vi "Camera_Feed.vi"(8 "error in":errorcluster, 11 "DataCluster":T1={"Core"={"Current VI Reference"=refnum, "Close Panel on Exit?"=FALSE, "Exit"=FALSE, "Initialized?"=FALSE}, "Connections"={"cDAQ Therm"={"Task"="", "Connected"=FALSE, "Active"=FALSE}, "cDAQ Voltage"={"Task"="", "Connected"=FALSE, "Active"=FALSE}, "cDAQ ID"="", "Camera"={"Session"="", "Connected"=FALSE, "Active"=FALSE, "Placeholder"=refnum}, "PSU"={"Port"="", "Connected"=FALSE, "Active"=FALSE}}, "Data Acquisition"={"Setup"={"Label"="", "Operator"="", "Notes"="", "TempGrad"=0.0, "TargetTemp"=0.0, "Sample Volume"=1.0}, "Camera"={"Image"=refnum, "Save Image"=refnum, "Image Frequency"=20, "Rectangle"={"Left"=0, "Top"=0, "Right"=0, "Bottom"=0, "Rotation"=0.0}, "Calibration"={"Top Left"={"X"=0.0, "Y"=0.0}, "Top Right"={"X"=0.0, "Y"=0.0}, "Bottom Left"={"X"=0.0, "Y"=0.0}, "Bottom Right"={"X"=0.0, "Y"=0.0}, "Fixpoint"={"X"=0.0, "Y"=0.0}, "Scan Area"=0.0, "Fixpoint Area"=0.0, "Well Pixels"=[], "Valid"=FALSE}, "FocusPos"=0, "Display Mapping"=10}, "Thermistor"={"Sample Size"=0, "Calibration"={"B0.100"=[], "R25"=[], "c"=[], "State"=[], "V_S"=0.0, "R_S"=0.0}, "Timing Mode"=14713}, "Partition"={"Data"=[], "Cell Label"="", "Cell Color"=0, "Height"=10, "Width"=16, "Grid"=[]}, "Queue"={"Size"=0, "Queue"=refnum}, "Sample Rate"=0, "Active"=FALSE, "Ready"=FALSE, "Graph Mode"=0}, "Control"={"Sample Rate"=0, "PID gains"={"proportional gain (Kc)"=0.0, "integral time (Ti, min)"=0.0, "derivative time (Td, min)"=0.0}}} {"Control"."PID gains"."derivative time (Td, min)" format="%.3f"; "Control"."PID gains"."integral time (Ti, min)" format="%.3f"; "Control"."PID gains"."proportional gain (Kc)" format="%.3f"; "Control"."Sample Rate" min=1 max=20 step=1 format="%.0f Samples/sec"; "Data Acquisition"."Graph Mode" items=["Thermistor Temperature", "Camera Temperature"]; "Data Acquisition"."Thermistor"."Timing Mode" items=["Automatic"=16097, "High Resolution"=10195, "High Speed"=14712, "Best 50 Hz Rejection"=14713, "Best 60 Hz Rejection"=14714, "Custom"=10137]; "Data Acquisition"."Thermistor"."Calibration"."R_S" min=0.1 max=1000.0 format="%#_g kOhm"; "Data Acquisition"."Thermistor"."Calibration"."V_S" min=5.0 max=48.0 format="%#_g V"; "Data Acquisition"."Thermistor"."Calibration"."R25" min=0.1 max=1000.0 format="%#_g kOhm"; "Data Acquisition"."Thermistor"."Calibration"."B0.100" min=100.0 max=10000.0 format="%#_g K"; "Data Acquisition"."Thermistor"."Sample Size" min=1 max=200; "Data Acquisition"."Sample Rate" min=20 max=240 format="%.0f samples/min"; "Data Acquisition"."Queue"."Size" min=1 max=200; "Data Acquisition"."Camera"."Display Mapping" items=["Default"=10, "Most Significant Bits"=11, "Full Dynamic"=12, "Downshift"=13, "Given Range"=14, "90% Dynamic"=15, "Given Percent Range"=16]; "Data Acquisition"."Camera"."Calibration"."Fixpoint"."Y" format="%.2f"; "Data Acquisition"."Camera"."Calibration"."Fixpoint"."X" format="%.2f"; "Data Acquisition"."Camera"."Calibration"."Top Left"."Y" format="%.2f"; "Data Acquisition"."Camera"."Calibration"."Top Left"."X" format="%.2f"; "Data Acquisition"."Camera"."Calibration"."Top Right"."Y" format="%.2f"; "Data Acquisition"."Camera"."Calibration"."Top Right"."X" format="%.2f"; "Data Acquisition"."Camera"."Calibration"."Bottom Left"."Y" format="%.2f"; "Data Acquisition"."Camera"."Calibration"."Bottom Left"."X" format="%.2f"; "Data Acquisition"."Camera"."Calibration"."Bottom Right"."Y" format="%.2f"; "Data Acquisition"."Camera"."Calibration"."Bottom Right"."X" format="%.2f"; "Data Acquisition"."Camera"."Rectangle"."Rotation" min=-90.0 max=90.0 step=1.0 format="%.2f"; "Data Acquisition"."Camera"."Rectangle"."Left" scale=0.0..1024.0; "Data Acquisition"."Camera"."Rectangle"."Right" scale=0.0..1024.0; "Data Acquisition"."Camera"."Image Frequency" min=1 max=60 step=1; "Data Acquisition"."Setup"."Sample Volume" min=0.0 max=500.0 format="%#_g µL"; "Data Acquisition"."Setup"."TargetTemp" min=-40.0 max=40.0 step=0.5 format="%#_g °C"; "Data Acquisition"."Setup"."TempGrad" min=-100.0 max=100.0 step=0.1 format="%#_g °C/min"}) -> (0 "error out":errorcluster, 3 "DataCluster out":T1={"Core"={"Current VI Reference"=refnum, "Close Panel on Exit?"=FALSE, "Exit"=FALSE, "Initialized?"=FALSE}, "Connections"={"cDAQ Therm"={"Task"="", "Connected"=FALSE, "Active"=FALSE}, "cDAQ Voltage"={"Task"="", "Connected"=FALSE, "Active"=FALSE}, "cDAQ ID"="", "Camera"={"Session"="", "Connected"=FALSE, "Active"=FALSE, "Placeholder"=refnum}, "PSU"={"Port"="", "Connected"=FALSE, "Active"=FALSE}}, "Data Acquisition"={"Setup"={"Label"="", "Operator"="", "Notes"="", "TempGrad"=1.0, "TargetTemp"=1.0, "Sample Volume"=1.0}, "Camera"={"Image"=refnum, "Save Image"=refnum, "Image Frequency"=20, "Rectangle"={"Left"=0, "Top"=0, "Right"=0, "Bottom"=0, "Rotation"=0.0}, "Calibration"={"Top Left"={"X"=0.0, "Y"=0.0}, "Top Right"={"X"=0.0, "Y"=0.0}, "Bottom Left"={"X"=0.0, "Y"=0.0}, "Bottom Right"={"X"=0.0, "Y"=0.0}, "Fixpoint"={"X"=0.0, "Y"=0.0}, "Scan Area"=0.0, "Fixpoint Area"=0.0, "Well Pixels"=[], "Valid"=FALSE}, "FocusPos"=0, "Display Mapping"=10}, "Thermistor"={"Sample Size"=1, "Calibration"={"B0.100"=[], "R25"=[], "c"=[], "State"=[], "V_S"=5.0, "R_S"=100.0}, "Timing Mode"=14713}, "Partition"={"Data"=[], "Cell Label"="", "Cell Color"=0, "Height"=10, "Width"=16, "Grid"=[]}, "Queue"={"Size"=1, "Queue"=refnum}, "Sample Rate"=20, "Active"=FALSE, "Ready"=FALSE, "Graph Mode"=0}, "Control"={"Sample Rate"=1, "PID gains"={"proportional gain (Kc)"=1.0, "integral time (Ti, min)"=0.01, "derivative time (Td, min)"=0.0}}} {"Control"."PID gains"."derivative time (Td, min)" format="%.3f"; "Control"."PID gains"."integral time (Ti, min)" format="%.3f"; "Control"."PID gains"."proportional gain (Kc)" format="%.3f"; "Control"."Sample Rate" min=1 max=20 step=1 format="%.0f Samples/sec"; "Data Acquisition"."Graph Mode" items=["Thermistor Temperature", "Camera Temperature"]; "Data Acquisition"."Thermistor"."Timing Mode" items=["Automatic"=16097, "High Resolution"=10195, "High Speed"=14712, "Best 50 Hz Rejection"=14713, "Best 60 Hz Rejection"=14714, "Custom"=10137]; "Data Acquisition"."Thermistor"."Calibration"."R_S" min=0.1 max=1000.0 format="%#_g kOhm"; "Data Acquisition"."Thermistor"."Calibration"."V_S" min=5.0 max=48.0 format="%#_g V"; "Data Acquisition"."Thermistor"."Calibration"."R25" min=0.1 max=1000.0 format="%#_g kOhm"; "Data Acquisition"."Thermistor"."Calibration"."B0.100" min=100.0 max=10000.0 format="%#_g K"; "Data Acquisition"."Thermistor"."Sample Size" min=1 max=200; "Data Acquisition"."Sample Rate" min=20 max=240 format="%.0f samples/min"; "Data Acquisition"."Queue"."Size" min=1 max=200; "Data Acquisition"."Camera"."Display Mapping" items=["Default"=10, "Most Significant Bits"=11, "Full Dynamic"=12, "Downshift"=13, "Given Range"=14, "90% Dynamic"=15, "Given Percent Range"=16]; "Data Acquisition"."Camera"."Calibration"."Fixpoint"."Y" format="%.2f"; "Data Acquisition"."Camera"."Calibration"."Fixpoint"."X" format="%.2f"; "Data Acquisition"."Camera"."Calibration"."Top Left"."Y" format="%.2f"; "Data Acquisition"."Camera"."Calibration"."Top Left"."X" format="%.2f"; "Data Acquisition"."Camera"."Calibration"."Top Right"."Y" format="%.2f"; "Data Acquisition"."Camera"."Calibration"."Top Right"."X" format="%.2f"; "Data Acquisition"."Camera"."Calibration"."Bottom Left"."Y" format="%.2f"; "Data Acquisition"."Camera"."Calibration"."Bottom Left"."X" format="%.2f"; "Data Acquisition"."Camera"."Calibration"."Bottom Right"."Y" format="%.2f"; "Data Acquisition"."Camera"."Calibration"."Bottom Right"."X" format="%.2f"; "Data Acquisition"."Camera"."Rectangle"."Rotation" min=-90.0 max=90.0 step=1.0 format="%.2f"; "Data Acquisition"."Camera"."Rectangle"."Left" scale=0.0..1024.0; "Data Acquisition"."Camera"."Rectangle"."Right" scale=0.0..1024.0; "Data Acquisition"."Camera"."Image Frequency" min=1 max=60 step=1; "Data Acquisition"."Setup"."Sample Volume" min=0.0 max=500.0 format="%#_g µL"; "Data Acquisition"."Setup"."TargetTemp" min=-40.0 max=40.0 step=0.5 format="%#_g °C"; "Data Acquisition"."Setup"."TempGrad" min=-100.0 max=100.0 step=0.1 format="%#_g °C/min"})   [LabVIEW 2020]
uses:
  DataCluster.ctl
  <vilib>/userDefined/High Color/IMAQdx.ctl
  <vilib>/vision/Image Controls.llb/IMAQ Image.ctl
  <resource>/objmgr/imaqdx.rc
panel:
  out "Feed":T3(plugin-control) caption="Camera Feed"
  out "FocusPos":u32 caption="Focus Position"
  in  "Autofocus":bool
  in  "Cropping":enum32{"Cropped", "Uncropped"}(radio)=enum."Uncropped"
  out "StatusString":string="Closing System"
  # "Select Region of Interest on the camera feed and see the  cropped image by selecting Cropped.\n\nMake sure the entire plate is within the boundaries"
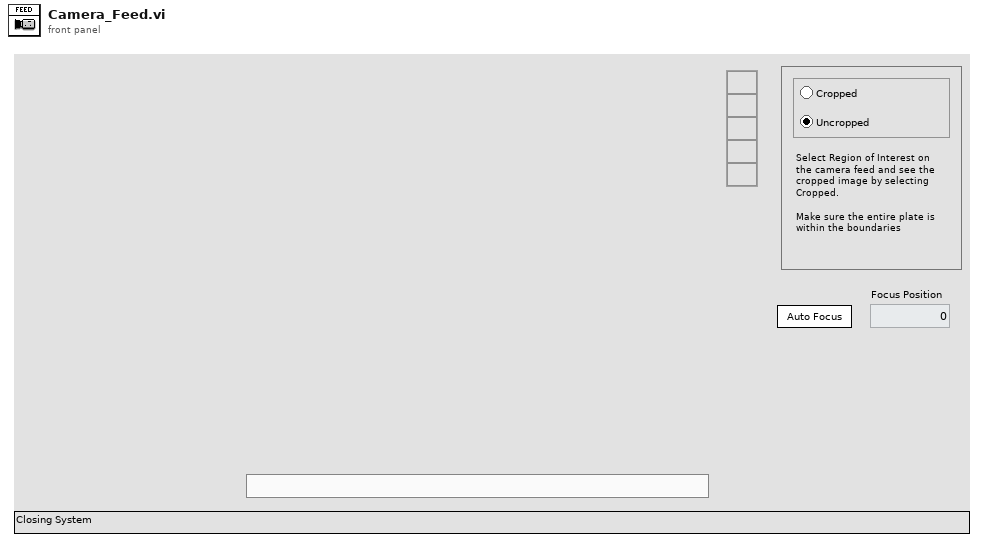
[diagram p1: front panel]
types:
  T1 = typedef "DataCluster.ctl" = cluster{"Core":cluster{"Current VI Reference":refnum<vi>, "Close Panel on Exit?":bool, "Exit":bool, "Initialized?":bool}, "Connections":cluster{"cDAQ Therm":cluster{"Task":refnum<k21>, "Connected":bool, "Active":bool}, "cDAQ Voltage":cluster{"Task":refnum<k21>, "Connected":bool, "Active":bool}, "cDAQ ID":string, "Camera":cluster{"Session":T2, "Connected":bool, "Active":bool, "Placeholder":T3}, "PSU":cluster{"Port":refnum<visa-resource-name>, "Connected":bool, "Active":bool}}, "Data Acquisition":cluster{"Setup":cluster{"Label":string, "Operator":string, "Notes":string, "TempGrad":dbl, "TargetTemp":dbl, "Sample Volume":dbl}, "Camera":cluster{"Image":T3, "Save Image":T3, "Image Frequency":i32, "Rectangle":T4, "Calibration":cluster{"Top Left":T5, "Top Right":T5, "Bottom Left":T5, "Bottom Right":T5, "Fixpoint":T5, "Scan Area":dbl, "Fixpoint Area":dbl, "Well Pixels":cluster{"X":i32, "Y":i32}[][], "Valid":bool}, "FocusPos":u32, "Display Mapping":u32}, "Thermistor":cluster{"Sample Size":i32, "Calibration":cluster{"B0.100":dbl[], "R25":dbl[], "c":dbl[][], "State":bool[], "V_S":dbl, "R_S":dbl}, "Timing Mode":i32}, "Partition":cluster{"Data":string[][], "Cell Label":string, "Cell Color":u32, "Height":i32, "Width":i32, "Grid":string[][]}, "Queue":cluster{"Size":i32, "Queue":refnum<queue>}, "Sample Rate":i32, "Active":bool, "Ready":bool, "Graph Mode":u16}, "Control":cluster{"Sample Rate":i32, "PID gains":cluster{"proportional gain (Kc)":dbl, "integral time (Ti, min)":dbl, "derivative time (Td, min)":dbl}}}
  T2 = typedef "IMAQdx.ctl" = refnum<k21>
  T3 = typedef "IMAQ Image.ctl" = refnum<image>
  T4 = typedef "IMAQ Rectangle" = cluster{"Left":i32, "Top":i32, "Right":i32, "Bottom":i32, "Rotation":dbl}
  T5 = typedef "IMAQ Point" = cluster{"X":sgl, "Y":sgl}
  T6 = enum32{"Invalid", "Standard", "Closed", "Hidden", "Minimized", "Maximized"}
  T7 = enum8{"Enabled", "Disabled", "Disabled and Grayed Out"}
  T8 = cluster{"Global Rectangle":i32[], "Contours":cluster{"Contour Type":u32, "ROI Type":u32, "Points":i32[]}[]}
  T9 = typedef "ROI Descriptor" = cluster{"Global Rectangle":i32[], "Contours":cluster{"ID":enum32{"External", "Internal"}, "Type":u32, "Coordinates":i32[]}[]}
  T10 = cluster{"Global Rectangle":i32[], "Contours":cluster{"Contour Type":u32, "Type":u32, "Coordinates":i32[]}[]}
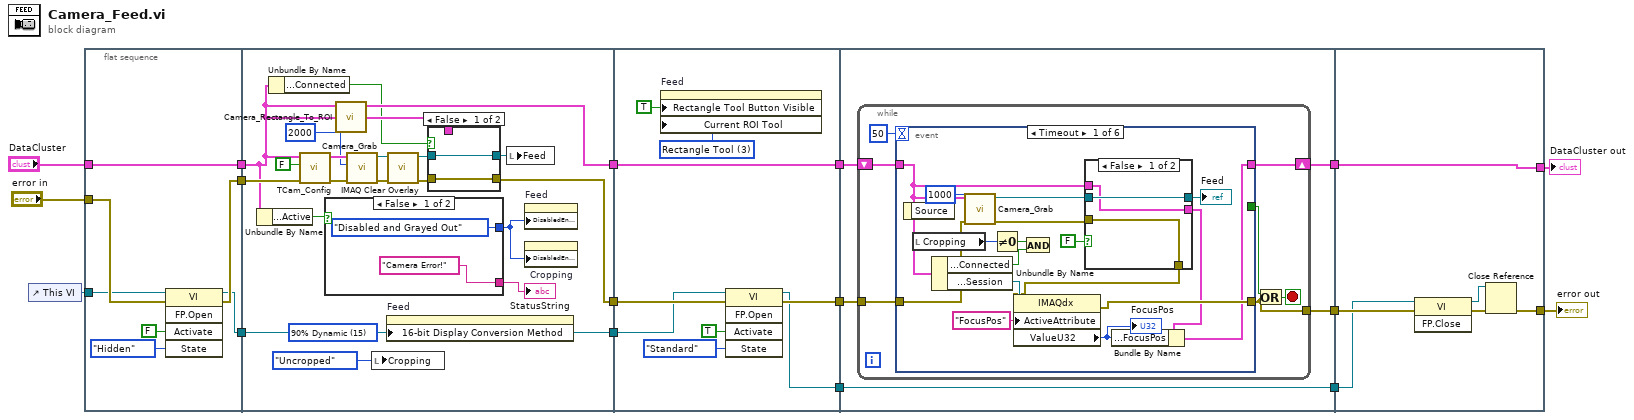
[diagram p0: block diagram]
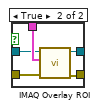
[diagram p2: hidden frame]
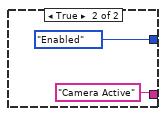
[diagram p3: hidden frame]
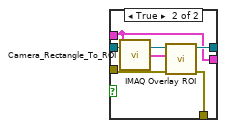
[diagram p4: hidden frame]
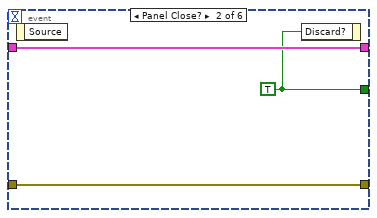
[diagram p5: hidden frame]
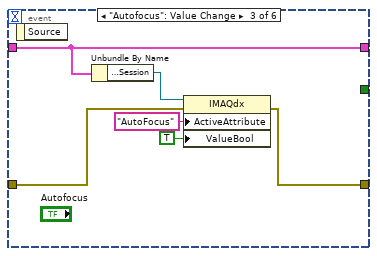
[diagram p6: hidden frame]
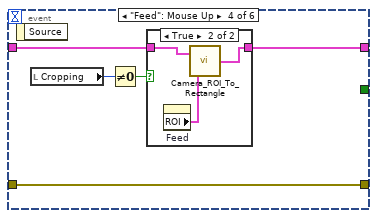
[diagram p7: hidden frame]
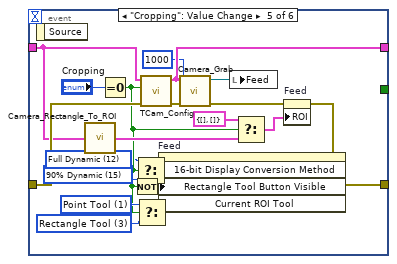
[diagram p9: hidden frame]
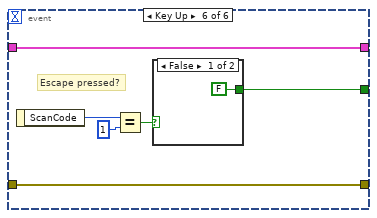
[diagram p10: hidden frame]
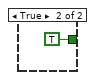
[diagram p11: hidden frame]
diagram:
  n1 = control-ref of="This VI"() -> (w3:refnum<vi>)
  n2 = flat-sequence {
    tunnel: "DataCluster" -> [w24]
    tunnel: "error in" -> [w23]
    tunnel: [w24] -> w7
    tunnel: w3 -> [w22]
    tunnel: [w20] -> w6
    tunnel: [w19] -> w4
    tunnel: [w37] -> w11
    tunnel: [w31] -> w9
    tunnel: w7 -> [w31]
    tunnel: w6 -> [w36]
    tunnel: [w35] -> w5
    tunnel: w4 -> [w35]
    tunnel: w11 -> [w61]
    tunnel: [w59] -> w10
    tunnel: w9 -> [w64]
    tunnel: [w64] -> w8
    tunnel: w5 -> [w60]
    tunnel: [w58] -> w1
    tunnel: [w67] -> w14
    tunnel: w10 -> [w69]
    tunnel: [w66] -> w13
    tunnel: w8 -> [w68]
    tunnel: [w65] -> w2
    tunnel: w1 -> [w65]
    tunnel: [w151] -> w15
    tunnel: w14 -> [w150]
    tunnel: [w154] -> w12
    tunnel: w13 -> [w154]
    tunnel: w2 -> [w149]
    frame #0 {
      n3 = invoke class="VI" method="FP.Open"(reference=w22, error in=w23, "Activate"=FALSE ("Activate?"), "State"=T6."Hidden") -> (reference out=w19:refnum<vi>, error out=w20:errorcluster)  [unwired: 1 in, 3 out]
    }
    frame #1 {
      w29 = u32 15 items=["Default"=10, "Most Significant Bits"=11, "Full Dynamic"=12, "Downshift"=13, "Given Range"=14, "90% Dynamic"=15, "Given Percent Range"=16] ("16-bit Display Mapping:Conversion Method")
      n4 = Unbundle By Name(w31) -> ("Connections.Camera.Active"=w43:bool)
      n5 = Unbundle By Name(w31) -> ("Connections.Camera.Connected"=w30:bool)
      n6 = call "TCam_Config.vi"("error in (no error)"=w36, "crop?"=FALSE, "DataCluster in"=w31) -> ("error out"=w38:errorcluster, "DataCluster out"=w39:T1)  [unwired: 7 in]
      n7 = case shown="False" w43 {
        tunnel: [T7."Disabled and Grayed Out" ("Disabled") T7."Enabled" ("Disabled")] -> w42
        tunnel: ["Camera Error!" "Camera Active"] -> w41
        frame False {
        }
        frame True {
        }
      }
      "StatusString" <- w41
      n8 = call "Camera_Rectangle_To_ROI.vi"("input cluster"=w31) -> ("ROI Descriptor"=w33:T9)
      n9 = call "Camera_Grab.vi"("error in"=w38, "Timeout (ms)"=2000, "DataCluster"=w39) -> ("error out"=w27:errorcluster, "Image Out"=w28:T3)  [unwired: 7 in]
      n10 = local write "Cropping"(enum32{"Cropped", "Uncropped"}."Uncropped" ("Cropping")) -> ()
      n11 = property on="Feed" class="ImageControl"("16-bit Display Conversion Method"=w29) -> ()  [unwired: 2 in, 2 out]
      n12 = call "IMAQ Clear Overlay"("error in (no error)"=w27, "Image"=w28) -> ("error out"=w26:errorcluster, "Image Out"=w25:T3)  [unwired: 8 in]
      n13 = case shown="False" w30 {
        tunnel: w25 -> [w45 w47]
        tunnel: w26 -> [w46 w48]
        tunnel: [w46 w51] -> w37
        tunnel: w33 -> [_ w50]
        tunnel: [w45 w49] -> w32
        frame False {
        }
        frame True {
          n14 = call "IMAQ Overlay ROI"("error in (no error)"=w48, "ROI Descriptor"=w50, "Image"=w47) -> ("error out"=w51:errorcluster, "Image Out"=w49:T3)  [unwired: 7 in]
        }
      }
      n15 = local write "Feed"(w32) -> ()
      n16 = property on="Feed" class="ImageControl"("DisabledEnum"=w42) -> ()  [unwired: 2 in, 2 out]
      n17 = property on="Cropping" class="RadioBtnsControl (strict)"("DisabledEnum"=w42) -> ()  [unwired: 2 in, 2 out]
    }
    frame #2 {
      w56 = u32 3 items=["Zoom Tool"=8, "Selection Tool"=0, "Pan Tool"=9, "Point Tool"=1, "Line Tool"=2, "Rectangle Tool"=3, "Rotated Rectangle Tool"=12, "Polyline Tool"=10, "Polygon Tool"=5, "Freehand Tool"=11, "Closed Freehand Tool"=6, "Ellipse Tool"=4, "Annulus Tool"=7] ("Current ROI Tool")
      n18 = property on="Feed" class="ImageControl"("Rectangle Tool Button Visible"=TRUE ("ROI Tool Buttons Visible:Rectangle Tool Button Visible"), "Current ROI Tool"=w56) -> ()  [unwired: 2 in, 2 out]
      n19 = invoke class="VI" method="FP.Open"(reference=w60, error in=w61, "Activate"=TRUE ("Activate?"), "State"=T6."Standard") -> (reference out=w58:refnum<vi>, error out=w59:errorcluster)  [unwired: 1 in, 3 out]
    }
    frame #3 {
      n20 = while {
        tunnel: w69 -> [w72]
        shift-right: [w74] -> w66
        shift-left: w68 -> [w73]
        tunnel: [w71] -> w67
        stop <- w75 stop-if-true
        n21 = event shown="[0] Timeout" {
          selector: _ -> [_ _ _ _ _ _]
          dyn-events: _ -> [_ _ _ _ _ _]
          timeout: 50 -> [_ _ _ _ _ _]
          tunnel: [_ w103 _ _ _ w146] -> w76
          tunnel: [w78 w105 w109 w116 w134 w142] -> w74
          tunnel: w73 -> [w85 w105 w109 w113 w131 w142]
          tunnel: w72 -> [w93 w104 w107 w112 w139 w141]
          tunnel: [w80 w104 w106 w112 w136 w141] -> w71
          event Timeout {
            n22 = event-data() -> ()  [unwired: 1 in, 1 out]
            n23 = local read "Cropping"() -> (w89:enum32{"Cropped", "Uncropped"})
            n24 = Unbundle By Name(w85) -> ("Connections.Camera.Connected"=w86:bool, "Connections.Camera.Session"=w82:T2)
            n25 = call "Camera_Grab.vi"("error in"=w93, "Timeout (ms)"=1000, "DataCluster"=w85) -> ("error out"=w90:errorcluster, "Image Out"=w91:T3)  [unwired: 7 in]
            n26 = Not Equal To 0?(x=w89) -> (x != 0?=w88:bool)
            n27 = And(x=w88, y=w86) -> ()  [unwired: 1 out]
            n28 = case shown="False" FALSE {
              tunnel: w91 -> [w96 w99]
              tunnel: w90 -> [w95 w98]
              tunnel: [w95 w102] -> w81
              tunnel: w85 -> [w94 w97]
              tunnel: [w96 w100] -> w87
              tunnel: [w94 w97] -> w79
              frame False {
              }
              frame True {
                n29 = call "Camera_Rectangle_To_ROI.vi"("input cluster"=w97) -> ("ROI Descriptor"=w101:T9)
                n30 = call "IMAQ Overlay ROI"("error in (no error)"=w98, "ROI Descriptor"=w101, "Image"=w99) -> ("error out"=w102:errorcluster, "Image Out"=w100:T3)  [unwired: 7 in]
              }
            }
            "Feed" <- w87
            n31 = property class="IMAQdx"(reference=w82, error in=w81, "ActiveAttribute"="FocusPos") -> (error out=w80:errorcluster, "ValueU32"=w77:u32)  [unwired: 1 out]
            "FocusPos" <- w77
            n32 = Bundle By Name(cluster=w79, "Data Acquisition.Camera.FocusPos"=w77) -> (w78:T1)
          }
          event Panel Close? {
            w103 = TRUE
            n33 = event-data() -> ()  [unwired: 1 in, 1 out]
            n34 = event-data("Discard?"=w103) -> ()  [unwired: 1 in, 1 out]
          }
          event "Autofocus": Value Change {
            n35 = event-data() -> ()  [unwired: 1 in, 1 out]
            n36 = Unbundle By Name(w109) -> ("Connections.Camera.Session"=w108:T2)
            n37 = property class="IMAQdx"(reference=w108, error in=w107, "ActiveAttribute"="AutoFocus", "ValueBool"=TRUE) -> (error out=w106:errorcluster)  [unwired: 1 out]
          }
          event "Feed": Mouse Up {
            n38 = event-data() -> ()  [unwired: 1 in, 1 out]
            n39 = local read "Cropping"() -> (w115:enum32{"Cropped", "Uncropped"})
            n40 = Not Equal To 0?(x=w115) -> (x != 0?=w114:bool)
            n41 = case shown="True" w114 {
              tunnel: [w117 w119] -> w116
              tunnel: w113 -> [w117 w120]
              frame False {
              }
              frame True {
                n42 = property on="Feed" class="ImageControl"() -> ("ROI"=w118:T8)  [unwired: 2 in, 2 out]
                n43 = call "Camera_ROI_To_Rectangle.vi"("ROI Descriptor"=w118, "input cluster"=w120) -> ("output cluster"=w119:T1)
              }
            }
          }
          event "Cropping": Value Change {
            w121 = u32 12 items=["Default"=10, "Most Significant Bits"=11, "Full Dynamic"=12, "Downshift"=13, "Given Range"=14, "90% Dynamic"=15, "Given Percent Range"=16] ("16-bit Display Mapping:Conversion Method")
            w122 = u32 15 items=["Default"=10, "Most Significant Bits"=11, "Full Dynamic"=12, "Downshift"=13, "Given Range"=14, "90% Dynamic"=15, "Given Percent Range"=16] ("16-bit Display Mapping:Conversion Method")
            w125 = u32 3 items=["Zoom Tool"=8, "Selection Tool"=0, "Pan Tool"=9, "Point Tool"=1, "Line Tool"=2, "Rectangle Tool"=3, "Rotated Rectangle Tool"=12, "Polyline Tool"=10, "Polygon Tool"=5, "Freehand Tool"=11, "Closed Freehand Tool"=6, "Ellipse Tool"=4, "Annulus Tool"=7] ("Current ROI Tool")
            w127 = u32 1 items=["Zoom Tool"=8, "Selection Tool"=0, "Pan Tool"=9, "Point Tool"=1, "Line Tool"=2, "Rectangle Tool"=3, "Rotated Rectangle Tool"=12, "Polyline Tool"=10, "Polygon Tool"=5, "Freehand Tool"=11, "Closed Freehand Tool"=6, "Ellipse Tool"=4, "Annulus Tool"=7] ("Current ROI Tool")
            n44 = event-data() -> ()  [unwired: 1 in, 1 out]
            n45 = call "Camera_Rectangle_To_ROI.vi"("input cluster"=w131) -> ("ROI Descriptor"=w130:T9)
            n46 = Equal To 0?(x="Cropping") -> (x = 0?=w123:bool)
            n47 = Not(x=w123) -> (.not. x?=w128:bool)
            n48 = Select(t=w121, s=w123, f=w122) -> (s? t:f=w124:u32)
            n49 = Select(t=w127, s=w123, f=w125) -> (s? t:f=w126:u32)
            n50 = call "TCam_Config.vi"("error in (no error)"=w139, "crop?"=w123, "DataCluster in"=w131) -> ("error out"=w135:errorcluster, "DataCluster out"=w134:T1)  [unwired: 7 in]
            n51 = property on="Feed" class="ImageControl"("16-bit Display Conversion Method"=w124, "Rectangle Tool Button Visible"=w128, "Current ROI Tool"=w126) -> ()  [unwired: 2 in, 2 out]
            n52 = call "Camera_Grab.vi"("error in"=w135, "Timeout (ms)"=1000, "DataCluster"=w134) -> ("error out"=w129:errorcluster, "Image Out"=w133:T3)  [unwired: 7 in]
            n53 = local write "Feed"(w133) -> ()
            n54 = Select(t=T8 {"Global Rectangle"=[], "Contours"=[]} ("ROI"), s=w123, f=w130) -> (s? t:f=w138:T10)
            n55 = property on="Feed" class="ImageControl"(error in=w129, "ROI"=w138) -> (error out=w136:errorcluster)  [unwired: 1 in, 1 out]
          }
          event Key Up {
            # "Escape pressed?"
            n56 = event-data() -> ("ScanCode"=w145:i16)  [unwired: 1 in]
            n57 = Equal?(x=w145, y=i16 1) -> (x = y?=w143:bool)
            n58 = case shown="False" w143 {
              tunnel: [FALSE TRUE] -> w146
              frame False {
              }
              frame True {
              }
            }
          }
        }
        n59 = Or(x=w76, y=w71) -> (x .or. y?=w75:bool)
      }
    }
    frame #4 {
      n60 = invoke class="VI" method="FP.Close"(reference=w149, error in=w150) -> (reference out=w153:refnum<vi>, error out=w152:errorcluster)  [unwired: 1 in, 1 out]
      n61 = Close Reference(reference=w153, error in (no error)=w152) -> (error out=w151:errorcluster)
    }
  }
  "error out" <- w15
  "DataCluster out" <- w12
